vi "solar_excel File Read (All).vi"(4 "Truncate Empty Cells? (F)":bool, 6 "Visible? (F)":bool, 8 "error in (no error)":errorcluster, 11 "Excel Workbook (*.xlsx)":path) -> (0 "error out":errorcluster, 1 "Worksheets Cells":cluster{"Cells":string[][]}[](array[cluster]), 2 "Worksheets":string[](array[string]), 3 "dup Excel Workbook":path)   [LabVIEW 2018]
doc: "This returns all Worksheets from an Excel Workbook (*.xlsx)."
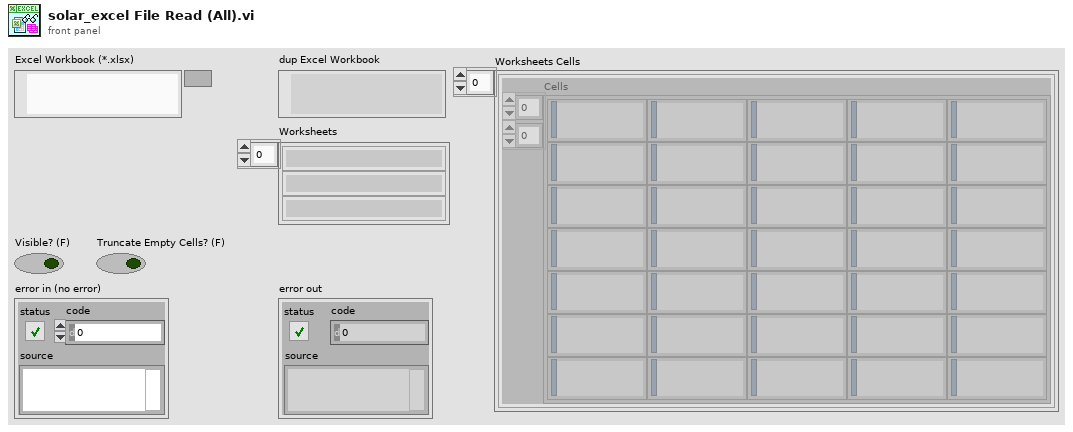
[diagram p1: front panel]
types:
  T1 = typedef "solar_excel_ctl App.ctl" = cluster{"ExcelApp":refnum<k7>, "Workbooks":refnum<k7>, "TSV":refnum<queue>}
  T2 = typedef "solar_excel_ctl Workbook.ctl" = cluster{"ExcelApp":refnum<k7>, "Workbooks":refnum<k7>, "TSV":refnum<queue>, "OpenWkb":refnum<k7>}
  T3 = typedef "solar_excel_ctl Worksheet.ctl" = cluster{"ExcelApp":refnum<k7>, "Workbooks":refnum<k7>, "TSV":refnum<queue>, "OpenWkb":refnum<k7>, "Worksheets":refnum<k7>, "OpenWksh":refnum<k7>}
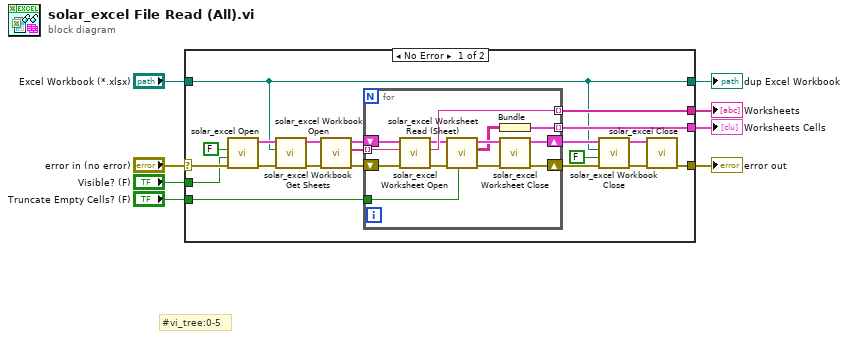
[diagram p0: block diagram]
diagram:
  # "#vi_tree:0-5"
  n1 = case shown="No Error" "error in (no error)" {
    selector: "error in (no error)" -> [w17 w43]
    tunnel: [w18 w43] -> w8
    tunnel: "Visible? (F)" -> [w16 _]
    tunnel: "Excel Workbook (*.xlsx)" -> [w9 w42]
    tunnel: [w13 _] -> w4
    tunnel: "Truncate Empty Cells? (F)" -> [w11 _]
    tunnel: [w10 _] -> w2
    tunnel: [w9 w42] -> w1
    frame No Error {
      n2 = call "solar_excel Open.vi"("error in (no error)"=w17, "Visible? (F)"=w16, "Open New Instance? (F)"=FALSE) -> ("error out"=w27:errorcluster, "Excel App"=w28:T1)  [unwired: 7 in]
      n3 = call "solar_excel Workbook Open.vi"("error in (no error)"=w27, "Excel Workbook (*.xlsx)"=w9, "Excel App"=w28) -> ("error out"=w26:errorcluster, "Excel Workbook"=w24:T2)  [unwired: 7 in]
      n4 = call "solar_excel Workbook Get Sheets.vi"("error in (no error)"=w26, "Excel Workbook in"=w24) -> ("error out"=w25:errorcluster, "Worksheet Names"=w15:string[], "Excel Workbook out"=w23:T2)  [unwired: 6 in, 1 out]
      n5 = for {
        tunnel: w15 -> [w37] mode=indexing
        shift-right: [w39] -> w22
        shift-left: w25 -> [w41]
        shift-right: [w38] -> w21
        shift-left: w23 -> [w40]
        tunnel: [w36] -> w13 mode=indexing
        tunnel: w11 -> [w32]
        tunnel: [w35] -> w10 mode=indexing
        n6 = call "solar_excel Worksheet Open.vi"("error in (no error)"=w41, "Sheet Name (STR) or Number (I32)"=w37, "Excel Workbook"=w40) -> ("error out"=w33:errorcluster, "Worksheet Name"=w35:string, "Excel Worksheet"=w34:T3)  [unwired: 5 in, 1 out]
        n7 = call "solar_excel Worksheet Read (Sheet).vi"("Truncate Empty Cells? (F)"=w32, "error in (no error)"=w33, "Excel Worksheet in"=w34) -> ("error out"=w30:errorcluster, "Cells"=w29:string[][], "Excel Worksheet out"=w31:T3)  [unwired: 6 in]
        n8 = Bundle("Cells"=w29) -> (w36:cluster{"Cells":string[][]})  [unwired: 1 in]
        n9 = call "solar_excel Worksheet Close.vi"("error in (no error)"=w30, "Excel Worksheet"=w31) -> ("error out"=w39:errorcluster, "Excel Workbook"=w38:T2)  [unwired: 8 in]
      }
      n10 = call "solar_excel Workbook Close.vi"("error in (no error)"=w22, "Save? (F)"=FALSE, "Excel Workbook (*.xlsx)"=w9, "Excel Workbook"=w21) -> ("error out"=w20:errorcluster, "Excel App"=w19:T1)  [unwired: 6 in]
      n11 = call "solar_excel Close.vi"("error in (no error)"=w20, "Excel App"=w19) -> ("error out"=w18:errorcluster)  [unwired: 9 in]
    }
    frame Error {
    }
  }
  "error out" <- w8
  "dup Excel Workbook" <- w1
  "Worksheets Cells" <- w4
  "Worksheets" <- w2
